vi "LOGIC_WaitNextFrame.vi"(8 "error in":errorcluster, 9 "index":u16, 10 "total buffers":u32, 11 "Database RefNum in":T1) -> (0 "error out":errorcluster, 2 "frame ready":T2)   [LabVIEW 2016]
uses:
  DBSHAND/private/vis/DatabaseHand_RefNum.ctl
panel:
  out "progress":u16
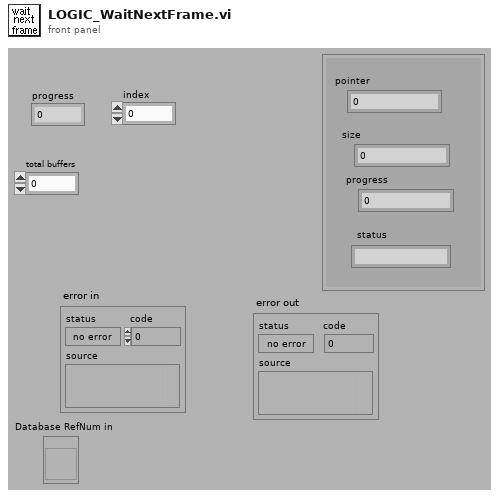
[diagram p1: front panel]
types:
  T1 = typedef "DatabaseHand_RefNum.ctl" = refnum<vi>
  T2 = cluster{"pointer":u64, "size":u64, "progress":u32, "status":string}
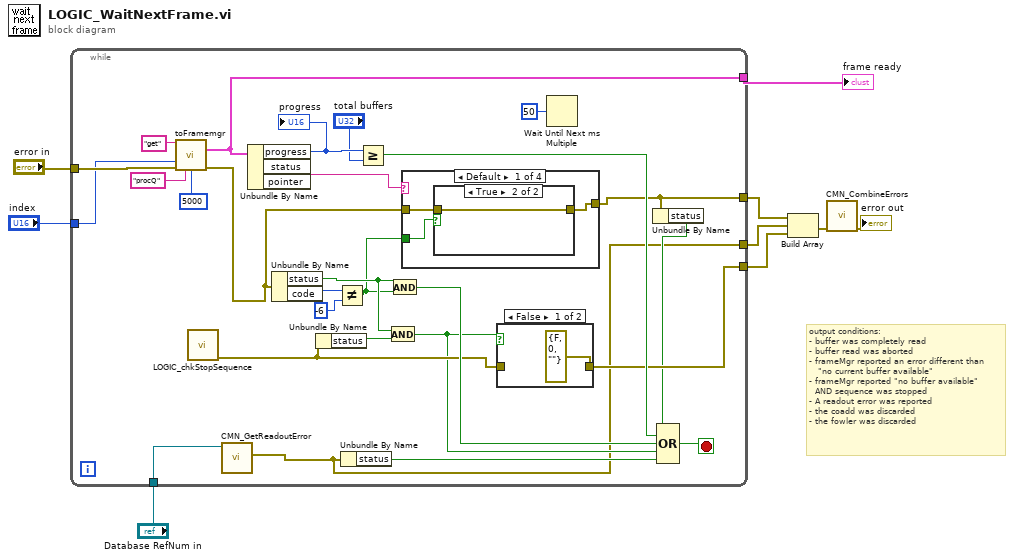
[diagram p0: block diagram]
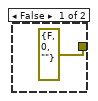
[diagram p3: hidden frame]
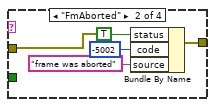
[diagram p4: hidden frame]
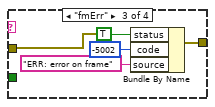
[diagram p5: hidden frame]
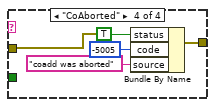
[diagram p6: hidden frame]
diagram:
  # "output conditions:\n- buffer was completely read\n- buffer read was aborted\n- frameMgr reported an error different than\n   \"no current buffer available\"\n- frameMgr reported \"no buffer available\"\n  AND sequence was stopped\n- A readout error was reported\n- the coadd was discarded\n- the fowler was discarded"
  n1 = while {
    tunnel: "index" -> [w12]
    tunnel: [w18] -> w3
    tunnel: [w11] -> w6
    tunnel: [w16] -> w7
    tunnel: "error in" -> [w29]
    tunnel: [w31] -> w9
    tunnel: "Database RefNum in" -> [w10]
    stop <- w27 stop-if-true
    n2 = call "toFramemgr.vi"("command"="get", "index"=w12, "error in"=w29, "responseQ"="procQ", "ms timeout (-1)"=5000) -> ("buffer"=w31:T2, "error out"=w25:errorcluster)  [unwired: 4 in, 5 out]
    n3 = call "LOGIC_chkStopSequence.vi"() -> ("error out"=w20:errorcluster)  [unwired: 11 out]
    n4 = call "CMN_GetReadoutError.vi"("Database RefNum in"=w10) -> ("readout_error"=w11:errorcluster)  [unwired: 1 in, 9 out]
    n5 = Unbundle By Name(w31) -> ("progress"=w33:u32, "status"=w17:string)  [unwired: 1 out]
    "progress" <- w33
    n6 = Unbundle By Name(w25) -> ("status"=w22:bool, "code"=w14:i32)
    n7 = Unbundle By Name(w20) -> ("status"=w23:bool)
    n8 = Not Equal?(x=w14, y=-6) -> (x != y?=w13:bool)
    n9 = Unbundle By Name(w11) -> ("status"=w21:bool)
    n10 = Greater Or Equal?(x=w33, y="total buffers") -> (x >= y?=w28:bool)
    n11 = And(x=w22, y=w23) -> (x .and. y?=w19:bool)
    n12 = And(x=w22, y=w13) -> (x .and. y?=w24:bool)
    n13 = case shown="Default" w17 {
      tunnel: w25 -> [w40 w44 w49 w54]
      tunnel: [w39 w45 w50 w55] -> w16
      tunnel: w13 -> [w41 _ _ _]
      frame Default {
        n14 = case shown="True" w41 {
          tunnel: w40 -> [_ w43]
          tunnel: [errorcluster {"status"=FALSE, "code"=0, "source"=""} ("error out") w43] -> w39
          frame False {
          }
          frame True {
          }
        }
      }
      frame "FmAborted" {
        n15 = Bundle By Name(cluster=w44, "status"=TRUE, "code"=-5002, "source"="frame was aborted") -> (w45:errorcluster)
      }
      frame "fmErr" {
        n16 = Bundle By Name(cluster=w49, "status"=TRUE, "code"=-5002, "source"="ERR: error on frame") -> (w50:errorcluster)
      }
      frame "CoAborted" {
        n17 = Bundle By Name(cluster=w54, "status"=TRUE, "code"=-5005, "source"="coadd was aborted") -> (w55:errorcluster)
      }
    }
    n18 = case shown="False" w19 {
      tunnel: w20 -> [_ w38]
      tunnel: [errorcluster {"status"=FALSE, "code"=0, "source"=""} ("error out") w38] -> w18
      frame False {
      }
      frame True {
      }
    }
    n19 = Wait Until Next ms Multiple(millisecond multiple=u32 50) -> ()  [unwired: 1 out]
    n20 = Unbundle By Name(w16) -> ("status"=w15:bool)
    n21 = Compound Arithmetic op=OR(w15, w28, w24, w19, w21) -> (w27:bool)
  }
  "frame ready" <- w9
  n22 = Build Array(w7, w6, w3) -> (w5:errorcluster[])
  n23 = call "CMN_CombineErrors.vi"("Errors"=w5) -> ("error out"=→"error out":errorcluster)  [unwired: 10 out]
